vi "Set Service map.vi"(10 "Service map":refnum<vi>, 11 "CANopen in":refnum<class "CANopen.lvclass">) -> (3 "CANopen out":refnum<class "CANopen.lvclass">)   [LabVIEW 2024]
uses:
  CANopen.lvclass/CANopen.ctl
  CANopen.lvclass
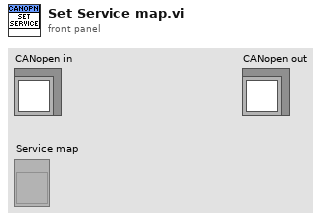
[diagram p1: front panel]
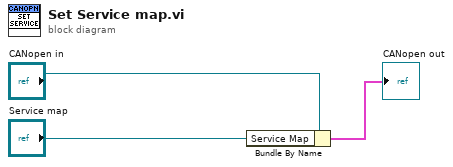
[diagram p0: block diagram]
diagram:
  n1 = Bundle By Name(cluster="CANopen in", "Service Map"="Service map") -> (→"CANopen out":cluster{})
